vi "F_conv_same.vi"(1 "dt":dbl=0.01, 2 "Pulse Pattern":dbl[](array[numeric])=array[50001 elements], 3 "Sinc Pattern":dbl[](array[numeric])=array[50001 elements]) -> (0 "Convolved":dbl[](array[numeric]))   [LabVIEW 2010]
uses:
  <vilib>/Analysis/2dsp.llb/1D Convolution (DBL).vi
  <vilib>/Analysis/NI_AALPro.lvlib
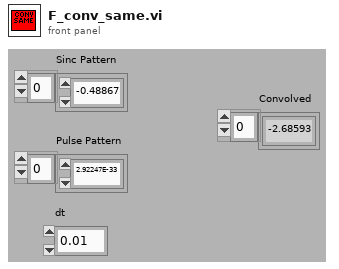
[diagram p1: front panel]
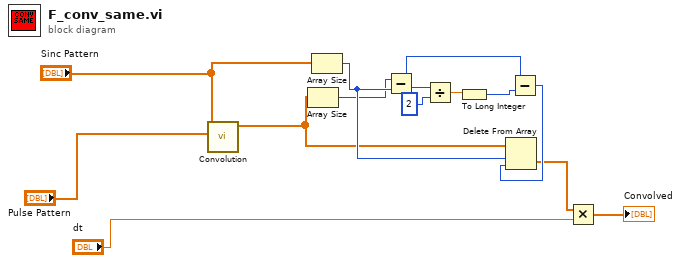
[diagram p0: block diagram]
diagram:
  n1 = call-poly <vilib>:"Convolution.vi"("Y"="Pulse Pattern", "X"="Sinc Pattern") -> ("X * Y"=w8:dbl[])  [unwired: 8 in, 1 out]
  n2 = Array Size(array=w8) -> (size(s)=w6:i32)
  n3 = Array Size(array="Sinc Pattern") -> (size(s)=w11:i32)
  n4 = Subtract(x=w6, y=w11) -> (x-y=w9:i32)
  n5 = Divide(x=w9, y=2) -> (x/y=w5:dbl)
  n6 = To Long Integer(number=w5) -> (32bit integer=w4:i32)
  n7 = Subtract(x=w9, y=w4) -> (x-y=w10:i32)
  n8 = Delete From Array(array=w8, length=w11, index=w10) -> (deleted portion=w3:dbl[])  [unwired: 1 out]
  n9 = Multiply(x=w3, y="dt") -> (x*y=→"Convolved":dbl[])
